vi "ASync-Resp TCP.vi"(7 "TcpRouter-Client in":refnum<class "TcpRouter-Client.lvclass">, 8 "error in (no error)":errorcluster) -> (0 "error out":errorcluster, 3 "connection ID":refnum<k5>)   [LabVIEW 2020, in "CSM-TCP-Router.lvlib" / "TcpRouter-Client.lvclass"]
uses:
  TcpRouter-Client.lvclass
  TcpRouter-Client.lvclass/TcpRouter-Client.ctl
  AsyncResp-Background-Thread.vi
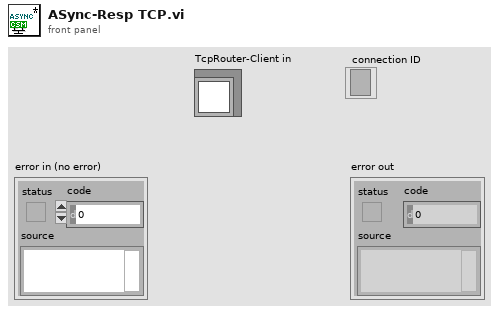
[diagram p1: front panel]
types:
  T1 = cluster{"IP Address":string, "Port":u16, "ConnectTMO":i32}
  T2 = typedef "CSM-TCP-Router.lvlib/TcpRouter-Client.lvclass/Def-TCP-Router ASYNC-RESP.ctl" = cluster{"Async-Resp":refnum<k5>, "RespQueue":refnum<queue>, "RespEvent":refnum<user-event>}
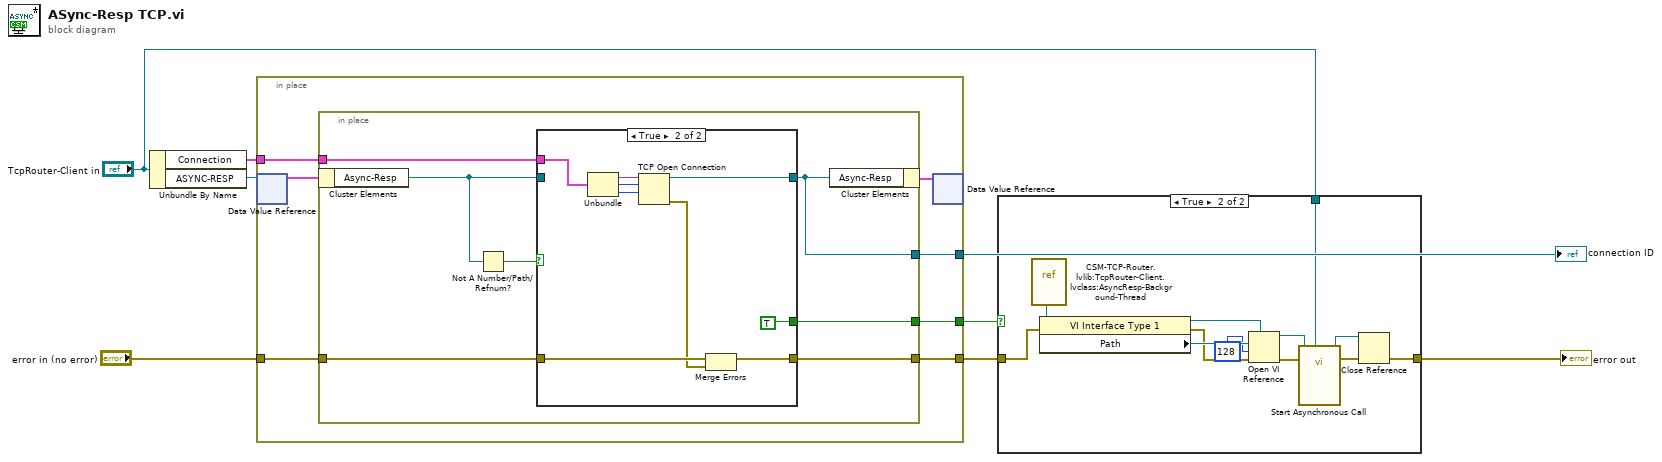
[diagram p0: block diagram]
diagram:
  n1 = Unbundle By Name("TcpRouter-Client in") -> ("Connection"=w6:T1, "ASYNC-RESP"=w7:refnum<data-value>)
  n2 = in-place {
    in-place-border: w6 -> [w13]
    in-place-border: [w12] -> w4
    in-place-border: "error in (no error)" -> [w11]
    in-place-border: [w10] -> w5
    in-place-border: [w9] -> w1
    n3 = in-place-dvr #1(w7) -> (w15:T2)  [unwired: 1 out]
    n4 = in-place {
      in-place-border: w13 -> [w22]
      in-place-border: [w20] -> w12
      in-place-border: w11 -> [w21]
      in-place-border: [w17] -> w10
      in-place-border: [w16] -> w9
      n5 = in-place-cluster #2(w15) -> ("Async-Resp"=w18:refnum<k5>)
      n6 = Not A Number/Path/Refnum?(number/path/refnum=w18) -> (NaN/Path/Refnum?=w19:bool)
      n7 = case shown="True" w19 {
        tunnel: w22 -> [_ w31]
        tunnel: w21 -> [w23 w30]
        tunnel: [w23 w29] -> w20
        tunnel: [w24 w27] -> w17
        tunnel: w18 -> [w24 _]
        tunnel: [_ TRUE] -> w16
        frame False {
        }
        frame True {
          n8 = Unbundle(w31) -> ("IP Address"=w33:string, "Port"=w32:u16, "ConnectTMO"=w26:i32)
          n9 = TCP Open Connection(address=w33, remote port or service name=w32, timeout ms (60000)=w26) -> (connection ID=w27:refnum<k5>, error out=w28:errorcluster)  [unwired: 2 in]
          n10 = Merge Errors(w30, w28) -> (w29:errorcluster)
        }
      }
      n11 = in-place-cluster #2("Async-Resp"=w17) -> (w14:T2)
    }
    n12 = in-place-dvr #1(w14) -> ()  [unwired: 2 out]
  }
  "connection ID" <- w5
  n13 = case shown="True" w1 {
    tunnel: [w34 w37] -> w3
    tunnel: w4 -> [w34 w36]
    tunnel: "TcpRouter-Client in" -> [_ w35]
    frame False {
    }
    frame True {
      n14 = vi-ref "CSM-TCP-Router.lvlib:TcpRouter-Client.lvclass:AsyncResp-Background-Thread.vi"() -> (w45:refnum<vi>)
      n15 = property class="VI Interface Type 1"(reference=w45, error in=w36) -> (reference out=w41:refnum<vi>, error out=w43:errorcluster, "Path"=w44:path)
      n16 = Open VI Reference(type specifier VI Refnum (for type only)=w41, vi path=w44, options=128, error in (no error)=w43) -> (vi reference=w42:refnum<vi>, error out=w46:errorcluster)  [unwired: 2 in]
      n17 = call-by-ref "Start Asynchronous Call"(reference=w42, error in=w46, "TcpRouter-Client"=w35) -> (reference out=w39:refnum<vi>, error out=w40:errorcluster)  [unwired: 10 in, 1 out]
      n18 = Close Reference(reference=w39, error in (no error)=w40) -> (error out=w37:errorcluster)
    }
  }
  "error out" <- w3
